vi "invers kinematic wire.vi"(0 "K":dbl, 7 "phi":dbl, 11 "s":dbl) -> (4 "L1":dbl, 8 "L 2":dbl, 15 "L 3":dbl)   [LabVIEW 2017]
uses:
  <vilib>/imath/engines/lvmath2/RunTimeEngine/Managers/WorkSpace/UID Generator.vi
  <vilib>/imath/engines/lvmath2/RunTimeEngine/RunTimeType/NIMS_RunTimeType_From StrictType (excl LVString).vi
  <instcachedir>/0/NIMS_RunTimeType_From StrictType (excl LVString)_1019F277F0A747EDBCA0F6C52CA54500.lvgen/NIMS_RunTimeType_From StrictType (excl LVString)_1019F277F0A747EDBCA0F6C52CA54500_000.vi
  <vilib>/imath/engines/lvmath2/RunTimeEngine/LocalVariableDefStatement/MC_LocalVariableDefStatement_Display.vi
  <vilib>/imath/engines/lvmath2/RunTimeEngine/Managers/SymbolTable/Clear UID.vi
  <vilib>/imath/engines/lvmath2/RunTimeEngine/NodeEndStatement/NIMS_NodeEndStatement_Output.vi
  <instcachedir>/0/NIMS_NodeEndStatement_Output_53EC0D466D134D7ABD903AC30B43404B.lvgen/NIMS_NodeEndStatement_Output_53EC0D466D134D7ABD903AC30B43404B_001.vi
  <vilib>/imath/engines/lvmath2/RunTimeEngine/ErrorHandling/NIMS_Finalize Error.vi
  <vilib>/imath/engines/lvmath2/RunTimeEngine/Managers/SymbolTable/NIMS_WorkSpace.lvlib
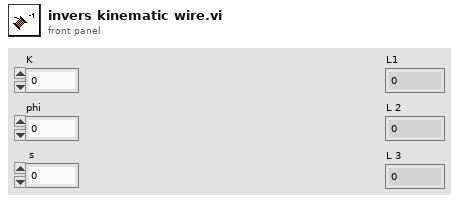
[diagram p1: front panel]
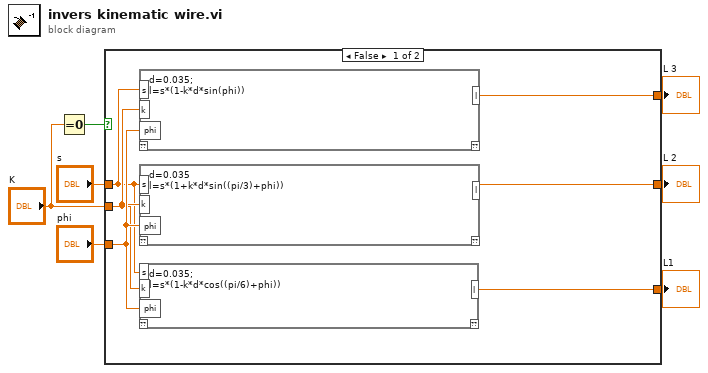
[diagram p0: block diagram]
diagram:
  n1 = Equal To 0?(x="K") -> (x = 0?=w7:bool)
  n2 = case shown="False" w7 {
    tunnel: [w13 w186] -> w6
    tunnel: "s" -> [w8 w186]
    tunnel: [w12 w186] -> w4
    tunnel: [w11 w186] -> w3
    tunnel: "K" -> [w9 _]
    tunnel: "phi" -> [w10 _]
    frame False {
      n3 = mathscript code="d=0.035;\nl=s*(1-k*d*sin(phi))"("s"=w8, "k"=w9, "phi"=w10) -> ("l"=w11:dbl)  [unwired: 1 in, 1 out]
      n4 = mathscript code="d=0.035\nl=s*(1+k*d*sin((pi/3)+phi))"("s"=w8, "k"=w9, "phi"=w10) -> ("l"=w12:dbl)  [unwired: 1 in, 1 out]
      n5 = mathscript code="d=0.035;\nl=s*(1-k*d*cos((pi/6)+phi))"("s"=w8, "k"=w9, "phi"=w10) -> ("l"=w13:dbl)  [unwired: 1 in, 1 out]
    }
    frame True {
    }
  }
  "L1" <- w6
  "L 2" <- w4
  "L 3" <- w3
